vi "Convert Data to DPIDs.vi"(8 "error in (no error)":errorcluster, 11 "Data":T1[](array[typedef]) {"payload" format="%x"; "timestamp" format="%<%.7X\n%x>T"; "type" items=["CAN Data"=0, "CAN Remote"=1, "CAN Bus Error"=2, "J1939 Data"=192, "Delay"=224, "Log Trigger"=225, "Start Trigger"=226]; "identifier" format="%x"}) -> (0 "error out":errorcluster, 1 "timestamp":timestamp, 2 "DPID Payload":u8[](array[numeric]), 3 "DPID ID":u8)   [LabVIEW 2015, in "GMLAN.lvlib"]
uses:
  GMLAN.lvlib
  <vilib>/xnet/xnet.llb/XNET Frame CAN.ctl
  <vilib>/xnet/xnet.llb/XNET Frame Type CAN.ctl
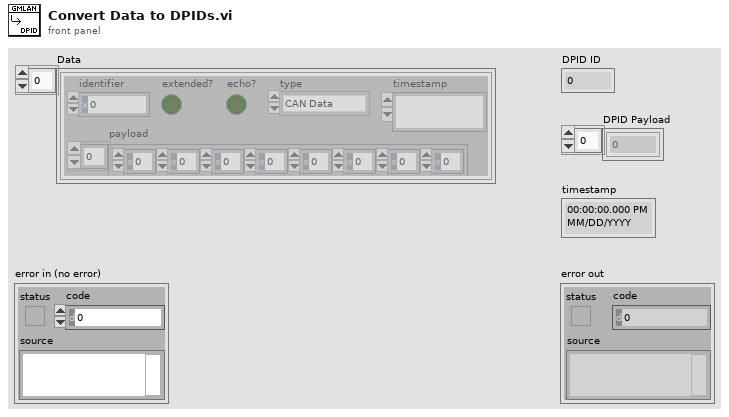
[diagram p1: front panel]
types:
  T1 = typedef "XNET Frame CAN.ctl" = cluster{"timestamp":timestamp, "payload":u8[], "identifier":u32, "type":T2, "extended?":bool, "echo?":bool}
  T2 = typedef "XNET Frame Type CAN.ctl" = u8
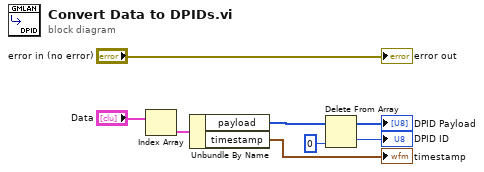
[diagram p0: block diagram]
diagram:
  n1 = Index Array(array="Data") -> (element=w7:T1)  [unwired: 1 in]
  n2 = Unbundle By Name(w7) -> ("payload"=w6:u8[], "timestamp"=→"timestamp":timestamp)
  n3 = Delete From Array(array=w6, index=0) -> (deleted portion=→"DPID ID":u8, array with subset deleted=→"DPID Payload":u8[])  [unwired: 1 in]
  "error out" <- "error in (no error)"
